vi "formatData.vi"(3 "error in (no error)":errorcluster, 4 "originalData":string, 5 "dataFormat":string) -> (0 "error out":errorcluster, 1 "formatedData":string)   [LabVIEW 2010]
panel:
  out "unsigned byte array":u8[](array[numeric])
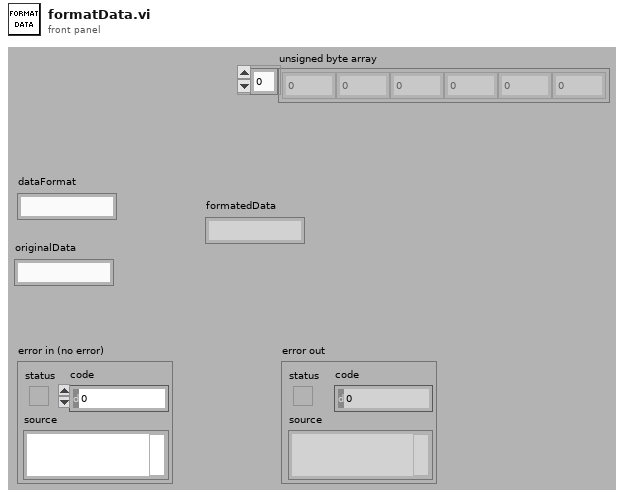
[diagram p1: front panel]
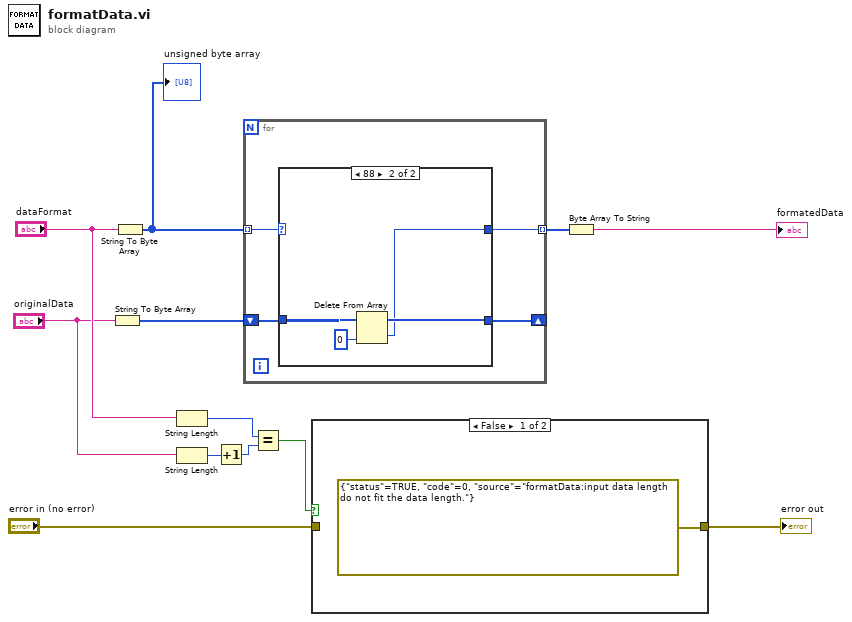
[diagram p0: block diagram]
diagram:
  n1 = String To Byte Array(string="originalData") -> (unsigned byte array=w11:u8[])
  n2 = String To Byte Array(string="dataFormat") -> (unsigned byte array=w12:u8[])
  "unsigned byte array" <- w12
  n3 = String Length(string="dataFormat") -> (length=w4:i32)
  n4 = String Length(string="originalData") -> (length=w6:i32)
  n5 = Increment(x=w6) -> (x+1=w5:i32)
  n6 = for {
    tunnel: w12 -> [w15] mode=indexing
    tunnel: [w16] -> w9 mode=indexing
    shift-right: [w13] -> _
    shift-left: w11 -> [w14]
    n7 = case shown="88" w15 {
      selector: w15 -> [w18 _]
      tunnel: [w18 w20] -> w16
      tunnel: w14 -> [w17 w22]
      tunnel: [w17 w21] -> w13
      frame 46, Default {
      }
      frame 88 {
        n8 = Delete From Array(array=w22, index=0) -> (deleted portion=w20:u8, array with subset deleted=w21:u8[])  [unwired: 1 in]
      }
    }
  }
  n9 = Equal?(x=w4, y=w5) -> (x = y?=w3:bool)
  n10 = case shown="False" w3 {
    tunnel: [errorcluster {"status"=TRUE, "code"=0, "source"="formatData:input data length do not fit the data length."} ("error out") w24] -> w2
    tunnel: "error in (no error)" -> [_ w24]
    frame False {
    }
    frame True {
    }
  }
  "error out" <- w2
  n11 = Byte Array To String(unsigned byte array=w9) -> (string=→"formatedData":string)
